vi "ALTS-2015 OPC Write LV2 Global.vi"(6 "OPC value Array":variant[](array[variant]), 7 "Options":T2, 8 "error in (no error)":errorcluster, 9 "OPC value":variant, 10 "OPC Write Register Array":T1[](array[typedef]), 11 "OPC Write Register":T1=enum."Serial_Flange_Size") -> (0 "error out":errorcluster, 2 "OPC Read Register Array Value":variant[](array[variant]), 3 "OPC Read Reigter Value":variant)   [LabVIEW 2013]
uses:
  Controls/ALTS-2015 OPC Write Global Options.ctl
  Controls/ALTS-2015 OPC Write Registers.ctl
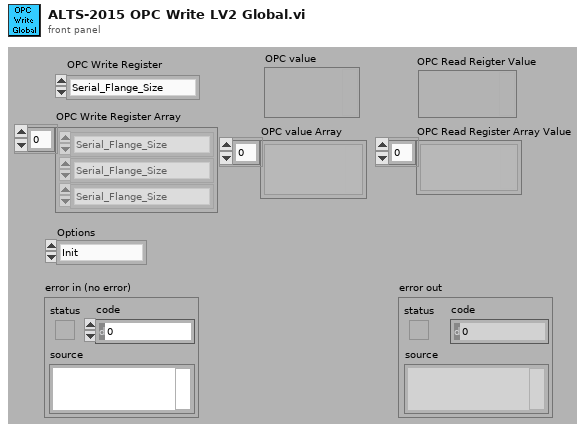
[diagram p1: front panel]
types:
  T1 = typedef "ALTS-2015 OPC Write Registers.ctl" = enum16{"Task_Available_for_Robot", "New_Serial", "Serial_Adapter_Size", "Serial_Displacement_Size", "Serial_Flange_Size", "Serial_Height", "Serial_LoadDecision", "Serial_CartInsert", "Test_Result", "Station_Number", "Rerun", "Invalid_SNo", "PC_ACK_Read_Tags", "No_Test"}
  T2 = typedef "ALTS-2015 OPC Write Global Options.ctl" = enum16{"Init", "Write Value", "Write Array", "Read Value", "Read Array", "Read All"}
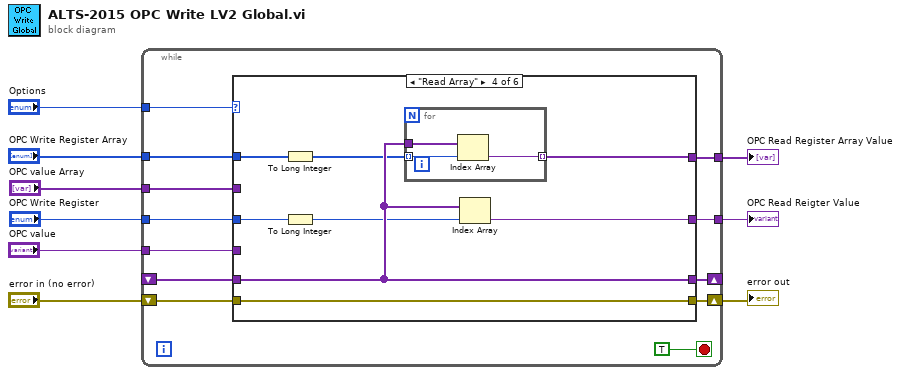
[diagram p0: block diagram]
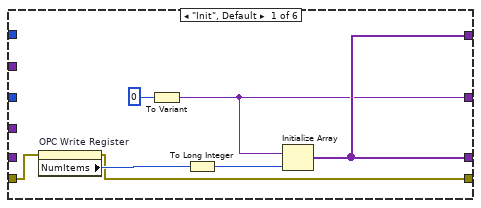
[diagram p2: hidden frame]
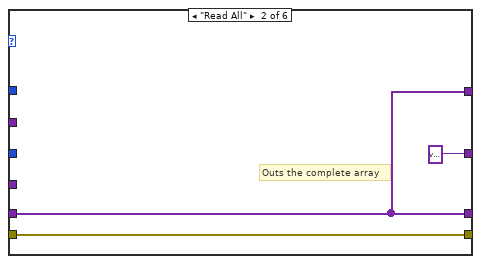
[diagram p3: hidden frame]
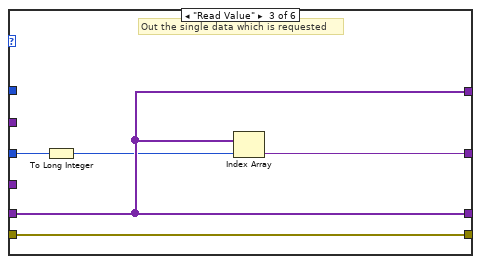
[diagram p4: hidden frame]
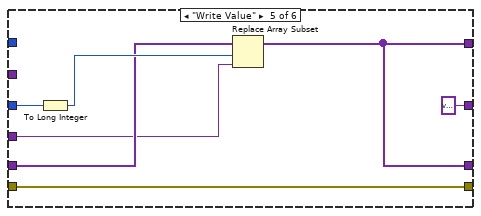
[diagram p5: hidden frame]
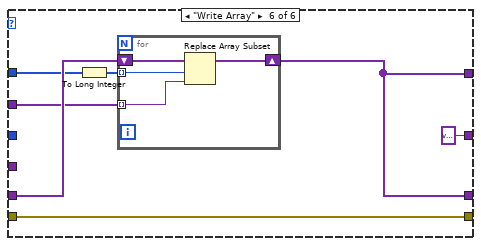
[diagram p6: hidden frame]
diagram:
  n1 = while {
    shift-right: [w20] -> _
    shift-left: _ -> [w19]
    tunnel: "OPC Write Register Array" -> [w18]
    tunnel: "OPC Write Register" -> [w17]
    tunnel: [w16] -> w7
    tunnel: [w15] -> w6
    shift-right: [w13] -> w4
    shift-left: "error in (no error)" -> [w14]
    tunnel: "OPC value Array" -> [w12]
    tunnel: "OPC value" -> [w11]
    tunnel: "Options" -> [w10]
    stop <- TRUE stop-if-true
    n2 = case shown="\"Read Array\"" w10 {
      tunnel: [w28 w31 w34 w41 w54 w58] -> w20
      tunnel: w19 -> [_ w31 w34 w41 w49 w57]
      tunnel: w18 -> [_ _ _ w44 _ w55]
      tunnel: w17 -> [_ _ w36 w40 w51 _]
      tunnel: [w22 variant ("OPC value") w35 w39 variant ("OPC value") variant ("OPC value")] -> w16
      tunnel: [w28 w31 w34 w43 w54 w58] -> w15
      tunnel: w14 -> [w26 w30 w33 w42 w53 w61]
      tunnel: [w25 w30 w33 w42 w53 w61] -> w13
      tunnel: w12 -> [_ _ _ _ _ w56]
      tunnel: w11 -> [_ _ _ _ w48 _]
      frame "Init", Default {
        n3 = property on="OPC Write Register" class="Enum (strict)"(error in=w26) -> (error out=w25:errorcluster, "NumItems"=w27:u32)  [unwired: 1 in, 1 out]
        n4 = To Variant(anything=0) -> (Variant=w22:variant)
        n5 = To Long Integer(number=w27) -> (32bit integer=w24:i32)
        n6 = Initialize Array(w22, w24) -> (w28:variant[])
      }
      frame "Read All" {
        # "Outs the complete array"
      }
      frame "Read Value" {
        # "Out the single data which is requested"
        n7 = To Long Integer(number=w36) -> (32bit integer=w32:i32)
        n8 = Index Array(array=w34, index=w32) -> (element=w35:variant)
      }
      frame "Read Array" {
        n9 = To Long Integer(number=w44) -> (32bit integer=w37:i32[])
        n10 = To Long Integer(number=w40) -> (32bit integer=w38:i32)
        n11 = for {
          tunnel: w41 -> [w47]
          tunnel: w37 -> [w46] mode=indexing
          tunnel: [w45] -> w43 mode=indexing
          n12 = Index Array(array=w47, index=w46) -> (element=w45:variant)
        }
        n13 = Index Array(array=w41, index=w38) -> (element=w39:variant)
      }
      frame "Write Value" {
        n14 = To Long Integer(number=w51) -> (32bit integer=w50:i32)
        n15 = Replace Array Subset(array=w49, new element=w48, index=w50) -> (w54:variant[])
      }
      frame "Write Array" {
        n16 = To Long Integer(number=w55) -> (32bit integer=w60:i32[])
        n17 = for {
          tunnel: w56 -> [w63] mode=indexing
          shift-right: [w64] -> w58
          shift-left: w57 -> [w65]
          tunnel: w60 -> [w62] mode=indexing
          n18 = Replace Array Subset(array=w65, new element=w63, index=w62) -> (w64:variant[])
        }
      }
    }
  }
  "error out" <- w4
  "OPC Read Reigter Value" <- w7
  "OPC Read Register Array Value" <- w6
